vi "Configure PointScan.vi"(0 "AODAcq in":refnum<class "AODAcq.lvclass">, 1 "Save":bool, 2 "Store Raw":bool, 5 "Points":i32[][](array[numeric]), 7 "GridSize":u32, 9 "Reps":u32, 11 "error in (no error)":errorcluster, 12 "Motion Points":u32, 14 "Motion Increment":u32) -> (4 "AODAcq out":refnum<class "AODAcq.lvclass">, 15 "error out":errorcluster)   [LabVIEW 2014, in "AODAcq.lvclass"]
uses:
  AODAcq.lvclass
  AODAcq.lvclass/AODAcq.ctl
  <vilib>/Utility/error.llb/Error Cluster From Error Code.vi
  C:/Program Files (x86)/National Instruments/LabVIEW 2014/Targets/NI/FPGA/StockFPGA_IntfPrivate/ScriptTemplates/StockFPGA_PlugInRead32.vi
  <vilib>/rvi/errors/niLvFpgaAdjustHostInterfaceError.vi
  HDF5Tools/LabView/Append To Dataset 2D Double.vi
  <vilib>/rvi/interface/nirviReadWriteControl/nirviReadWriteControl.xnode
  FPGA_Control/AODRef.ctl
  FPGA Bitfiles/AodScanner_FPGATarget_AODControl(FPGA)_TyJc9yYmyGA.lvbitx
  HDF5Tools/LabView/HDF5Tools.lvlib
  NiFpgaLv.dll
  <vilib>/FPGAPlugInAG/PXIe-7965R/niLvFpga_Read32_PXIe-7965R.vi
  <vilib>/rvi/interface/nirviReadWriteControl/niFpgaRWControlAccessTimeoutTemplate.vi
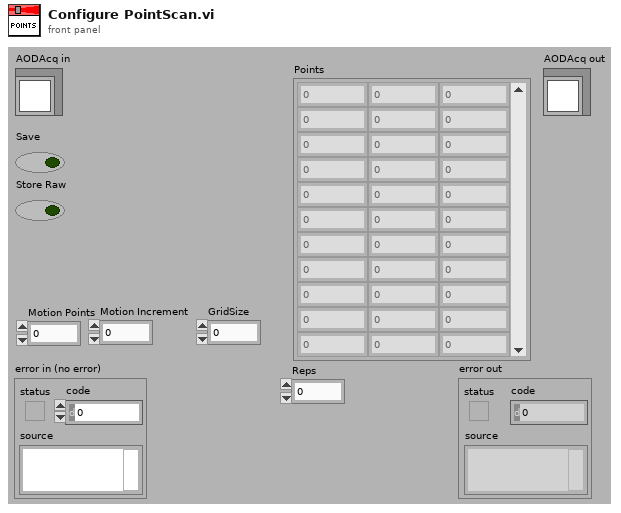
[diagram p1: front panel]
types:
  T1 = typedef "AODRef.ctl" = refnum<k20>
  T2 = cluster{"file handle out":i32, "ImData":i32, "TemporalData":i32, "MotionData":i32, "RawData":i32, "AODMotionCorrectionData":i32, "MotorMotionCorrectionData":i32, "MotionCoordinates":i32, "PointCoordinates":i32}
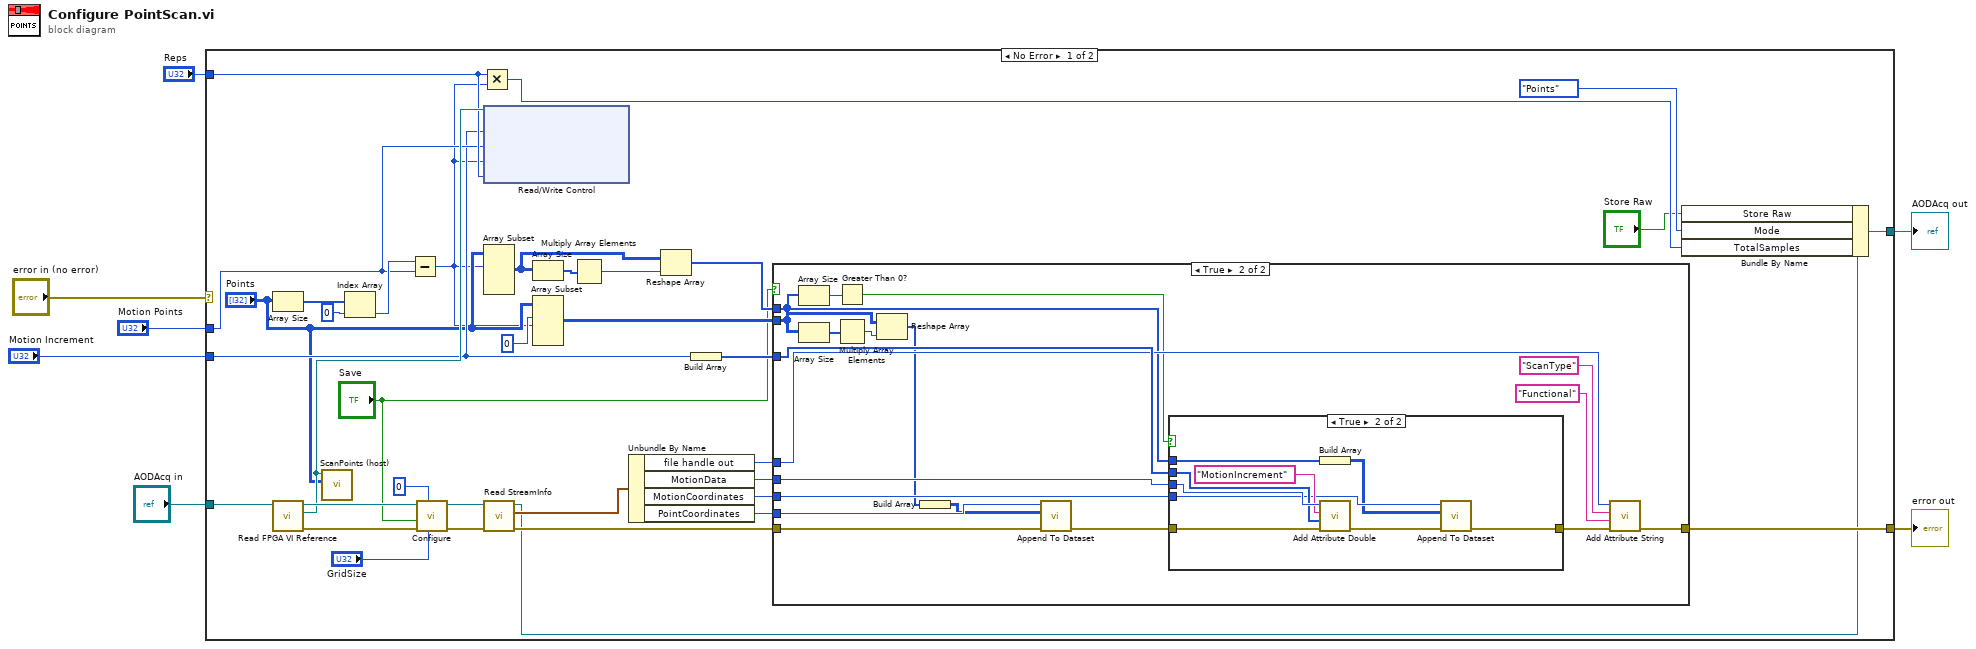
[diagram p0: block diagram]
diagram:
  n1 = case shown="No Error" "error in (no error)" {
    selector: "error in (no error)" -> [_ w75]
    tunnel: [w35 w75] -> w6
    tunnel: [w32 w74] -> w4
    tunnel: "AODAcq in" -> [w42 w74]
    tunnel: "Motion Increment" -> [w24 _]
    tunnel: "Motion Points" -> [w25 _]
    tunnel: "Reps" -> [w27 _]
    frame No Error {
      n2 = Array Size(array="Points") -> (size(s)=w34:i32[])
      n3 = call-dynamic "Read FPGA VI Reference.vi"("AODAcq in"=w42) -> ("error out"=w39:errorcluster, "FPGA VI Reference"=w29:T1, "AODAcq out"=w41:refnum<class "AODAcq.lvclass">)  [unwired: 8 in]
      n4 = call "ScanPoints (host).vi"("Points"="Points", "FPGA VI Reference Out"=w29) -> ()  [unwired: 10 in]
      n5 = Index Array(array=w34, index=0) -> (element=w28:i32)
      n6 = Subtract(x=w28, y=w25) -> (x-y=w18:u32)
      n7 = call-dynamic "Configure.vi"("GridSize"="GridSize", "Mode"=u32 0, "error in (no error)"=w39, "Save"="Save", "AODAcq in"=w41) -> ("error out"=w38:errorcluster, "AODAcq out"=w40:refnum<class "AODAcq.lvclass">)  [unwired: 5 in]
      n8 = Multiply(x=w27, y=w18) -> (x*y=w31:u32)
      n9 = xnode "Read/Write Control"("FPGA VI Reference In"=w29, "Scan.Motion Increment"=w24, "Scan.NumMotionPoints"=w25, "Scan.NumPoints"=w18, "Scan.NumReps"=w27) -> ()  [unwired: 1 in, 2 out]
      n10 = Array Subset(array="Points", index (row)=w18) -> (w15:i32[][])  [unwired: 3 in]
      n11 = call-dynamic "Read StreamInfo.vi"("error in (no error)"=w38, "AODAcq in"=w40) -> ("error out"=w36:errorcluster, "StreamInfo"=w37:T2, "AODAcq out"=w9:refnum<class "AODAcq.lvclass">)  [unwired: 7 in]
      n12 = Array Size(array=w15) -> (size(s)=w16:i32[])
      n13 = Array Subset(array="Points", index (row)=0 ("index"), length (row)=w18) -> (w20:i32[][])  [unwired: 2 in]
      n14 = Multiply Array Elements(1:w16) -> (0:w17:i32)
      n15 = Unbundle By Name(w37) -> ("file handle out"=w13:i32, "MotionData"=w23:i32, "MotionCoordinates"=w10:i32, "PointCoordinates"=w8:i32)
      n16 = Reshape Array(w15, w17) -> (w14:i32[])
      n17 = Build Array(w24) -> (w22:u32[])
      n18 = case shown="True" "Save" {
        tunnel: w20 -> [_ w61]
        tunnel: w36 -> [w44 w49]
        tunnel: [w44 w58] -> w35
        tunnel: w23 -> [_ w60]
        tunnel: w22 -> [_ w59]
        tunnel: w14 -> [_ w56]
        tunnel: w13 -> [_ w57]
        tunnel: w10 -> [_ w50]
        tunnel: w8 -> [_ w47]
        frame False {
        }
        frame True {
          n19 = Array Size(array=w56) -> (size(s)=w55:i32)
          n20 = Array Size(array=w61) -> (size(s)=w62:i32[])
          n21 = Greater Than 0?(x=w55) -> (x > 0?=w54:bool)
          n22 = Multiply Array Elements(1:w62) -> (0:w63:i32)
          n23 = Reshape Array(w61, w63) -> (w46:i32[])
          n24 = Build Array(w46) -> (w45:i32[][])
          n25 = call-poly "Append To Dataset.vi"("Error in (no error)"=w49, "Data"=w45, "Dataset id in"=w47) -> ("Error out"=w48:errorcluster)  [unwired: 7 in, 1 out]
          n26 = case shown="True" w54 {
            tunnel: w60 -> [_ w73]
            tunnel: w48 -> [w64 w72]
            tunnel: w59 -> [_ w71]
            tunnel: w56 -> [_ w66]
            tunnel: [w64 w67] -> w51
            tunnel: w50 -> [_ w69]
            frame False {
            }
            frame True {
              n27 = Build Array(w66) -> (w65:i32[][])
              n28 = call "Add Attribute Double.vi"("error in (no error)"=w72, "data"=w71, "Attribute name"="MotionIncrement", "loc_id"=w73) -> ("error out"=w68:errorcluster)  [unwired: 6 in, 1 out]
              n29 = call-poly "Append To Dataset.vi"("Error in (no error)"=w68, "Data"=w65, "Dataset id in"=w69) -> ("Error out"=w67:errorcluster)  [unwired: 7 in, 1 out]
            }
          }
          n30 = call "Add Attribute String.vi"("error in (no error)"=w51, "Attribute data"="Functional", "Attribute name"="ScanType", "loc_id"=w57) -> ("error out"=w58:errorcluster)  [unwired: 6 in, 1 out]
        }
      }
      n31 = Bundle By Name(cluster=w9, "Store Raw"="Store Raw", "Mode"=enum16{"Idle", "Points", "Volume"}."Points", "TotalSamples"=w31) -> (w32:refnum<class "AODAcq.lvclass">)
    }
    frame Error {
    }
  }
  "error out" <- w6
  "AODAcq out" <- w4
